vi "System IDs.vi"(11 "Node Config in":refnum<class "Node Config.lvclass">) -> (1 "Name":string, 2 "Cluster":string, 3 "System":string)   [LabVIEW 2020, in "Vecto.lvlib" / "Node Config.lvclass"]
uses:
  Node Config.lvclass
  Node Config.lvclass/Node Config.ctl
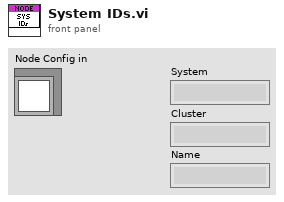
[diagram p1: front panel]
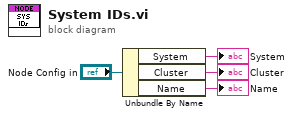
[diagram p0: block diagram]
diagram:
  n1 = Unbundle By Name("Node Config in") -> ("System"=→"System":string, "Cluster"=→"Cluster":string, "Name"=→"Name":string)
